vi "KH_DAQ_TURCK_DO_Count.vi"(8 "EIP_DI":T3 {"Nr" max=63; "Chan" max=63}, 10 "EIP_DO":T1 {"Nr" max=63; "Chan" max=63}, 11 "Config":T4[](array[typedef])) -> ()   [LabVIEW 2021]
uses:
  KH EthernetIPConfig 17.14/KH EthernetIPConfig TDef Config.ctl
  KH EthernetIPConfig 17.14/KH EthernetIPConfig TypeDefs ModuleTyp.ctl
  KH_DAQ_TURCK_TypeDefs_Cluster DI.ctl
  KH_DAQ_TURCK_TypeDefs_Cluster DO.ctl
  KH_DAQ_TURCK_Global.vi
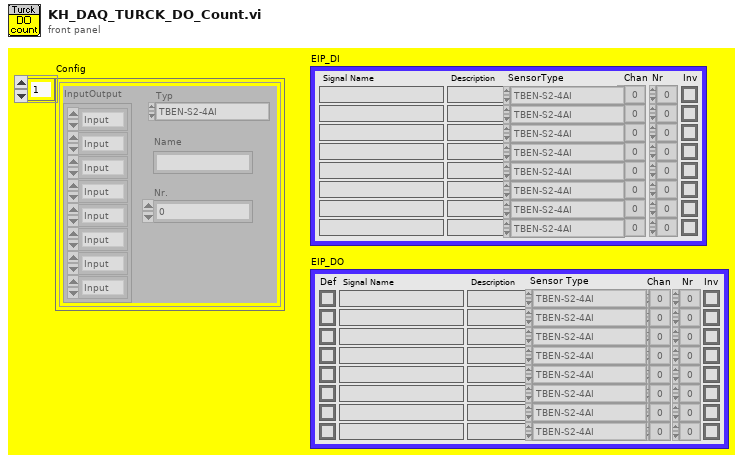
[diagram p1: front panel]
types:
  T1 = typedef "KH_DAQ_TURCK_TypeDefs_Cluster DO.ctl" = cluster{"Def":bool[], "Signal Name":string[], "Description":string[], "Chan":u16[], "Inv":bool[], "Nr":u16[], "SensorType":T2[]}
  T2 = typedef "KH EthernetIPConfig TypeDefs ModuleTyp.ctl" = enum16{"TBEN-S2-4AI", "TBEN-S1-8DXP", "TBEN-S2-2RFID-4DXP", "TBEN-S2-4AO", "TBEN-S2-4IOL"}
  T3 = typedef "KH_DAQ_TURCK_TypeDefs_Cluster DI.ctl" = cluster{"Signal Name":string[], "Description":string[], "Chan":u16[], "Inv":bool[], "Nr":u16[], "SensorType":T2[]}
  T4 = typedef "KH EthernetIPConfig TDef Config.ctl" = cluster{"Typ":T2, "Name":string, "Nr.":i32, "InputOutput":enum16{"Input", "Output"}[]}
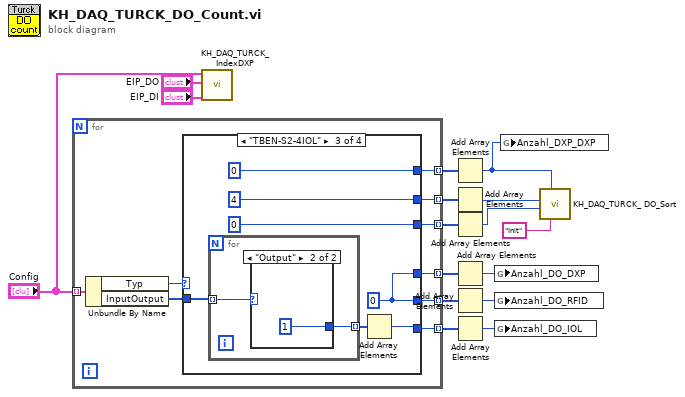
[diagram p0: block diagram]
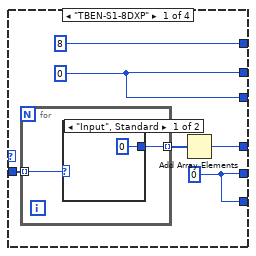
[diagram p2: hidden frame]
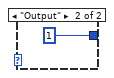
[diagram p3: hidden frame]
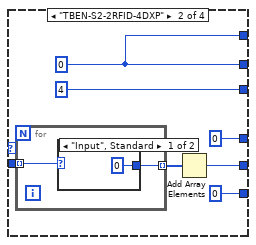
[diagram p4: hidden frame]
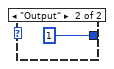
[diagram p5: hidden frame]
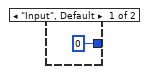
[diagram p6: hidden frame]
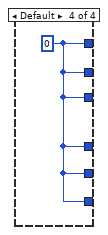
[diagram p7: hidden frame]
diagram:
  n1 = for {
    tunnel: "Config" -> [w25] mode=indexing
    tunnel: [w23] -> w16 mode=indexing
    tunnel: [w22] -> w15 mode=indexing
    tunnel: [w21] -> w14 mode=indexing
    tunnel: [w19] -> w13 mode=indexing
    tunnel: [w18] -> w10 mode=indexing
    tunnel: [w17] -> w9 mode=indexing
    n2 = Unbundle By Name(w25) -> ("Typ"=w24:T2, "InputOutput"=w20:enum16{"Input", "Output"}[])
    n3 = case shown="\"TBEN-S2-4IOL\"" w24 {
      tunnel: [8 w41 0 w58] -> w23
      tunnel: [w30 w41 4 w58] -> w22
      tunnel: [w30 4 0 w58] -> w21
      tunnel: w20 -> [w29 w39 w48 _]
      tunnel: [w26 0 w47 w58] -> w19
      tunnel: [w27 w40 w47 w58] -> w18
      tunnel: [w27 0 w50 w58] -> w17
      frame "TBEN-S1-8DXP" {
        w27 = 0
        w30 = 0
        n4 = for {
          tunnel: w29 -> [w33] mode=indexing
          tunnel: [w32] -> w28 mode=indexing
          n5 = case shown="\"Input\", Standard" w33 {
            tunnel: [0 1] -> w32
            frame "Input", Default {
            }
            frame "Output" {
            }
          }
        }
        n6 = Add Array Elements(numeric array=w28) -> (sum=w26:i32)
      }
      frame "TBEN-S2-2RFID-4DXP" {
        w41 = 0
        n7 = for {
          tunnel: w39 -> [w44] mode=indexing
          tunnel: [w43] -> w38 mode=indexing
          n8 = case shown="\"Input\", Standard" w44 {
            tunnel: [0 1] -> w43
            frame "Input", Default {
            }
            frame "Output" {
            }
          }
        }
        n9 = Add Array Elements(numeric array=w38) -> (sum=w40:i32)
      }
      frame "TBEN-S2-4IOL" {
        w47 = 0
        n10 = for {
          tunnel: w48 -> [w55] mode=indexing
          tunnel: [w54] -> w49 mode=indexing
          n11 = case shown="\"Output\"" w55 {
            tunnel: [0 1] -> w54
            frame "Input", Default {
            }
            frame "Output" {
            }
          }
        }
        n12 = Add Array Elements(numeric array=w49) -> (sum=w50:i32)
      }
      frame Default {
        w58 = 0
      }
    }
  }
  n13 = call "KH_DAQ_TURCK_IndexDXP.vi"("EIP_DI"="EIP_DI", "EIP_DO"="EIP_DO", "Config"="Config") -> ()  [unwired: 9 in]
  n14 = Add Array Elements(numeric array=w16) -> (sum=w2:i32)
  n15 = Add Array Elements(numeric array=w15) -> (sum=w5:i32)
  n16 = Add Array Elements(numeric array=w14) -> (sum=w4:i32)
  n17 = Add Array Elements(numeric array=w13) -> (sum=w12:i32)
  n18 = Add Array Elements(numeric array=w10) -> (sum=w11:i32)
  n19 = Add Array Elements(numeric array=w9) -> (sum=w8:i32)
  n20 = global write "KH_DAQ_TURCK_Global.vi" "Anzahl_DO_DXP"(w12) -> ()
  n21 = global write "KH_DAQ_TURCK_Global.vi" "Anzahl_DO_RFID"(w11) -> ()
  n22 = global write "KH_DAQ_TURCK_Global.vi" "Anzahl_DO_IOL"(w8) -> ()
  n23 = global write "KH_DAQ_TURCK_Global.vi" "Anzahl_DXP_DXP"(w2) -> ()
  n24 = call "KH_DAQ_TURCK_ DO_Sort.vi"("Function"="Init", "Anzahl_DXP_DXP"=w2, "Anzahl_DXP_RFID"=w4, "Anzahl_DXP_IOL"=w5) -> ()  [unwired: 4 in, 4 out]
